vi "update GUI KF tuning.vi"(10 "Supervisor in":refnum<class "Supervisor.lvclass">, 11 "Vessel in":refnum<class "Vessel.lvclass">) -> (2 "Supervisor":refnum<class "Supervisor.lvclass">)   [LabVIEW 2014]
uses:
  ROV/Vessel.lvclass
  Supervisor/Supervisor.lvclass
  <vilib>/Analysis/Matrix/Datatypes/RealMatrix.ctl
  Observer/Kalman Filter/Kalman Filter.lvclass
  <vilib>/Analysis/Matrix/NI_Matrix.lvlib
panel:
  out "Real Matrix":T1
  in  "Name":string
  in  "Update Q":bool
  in  "Update R":bool
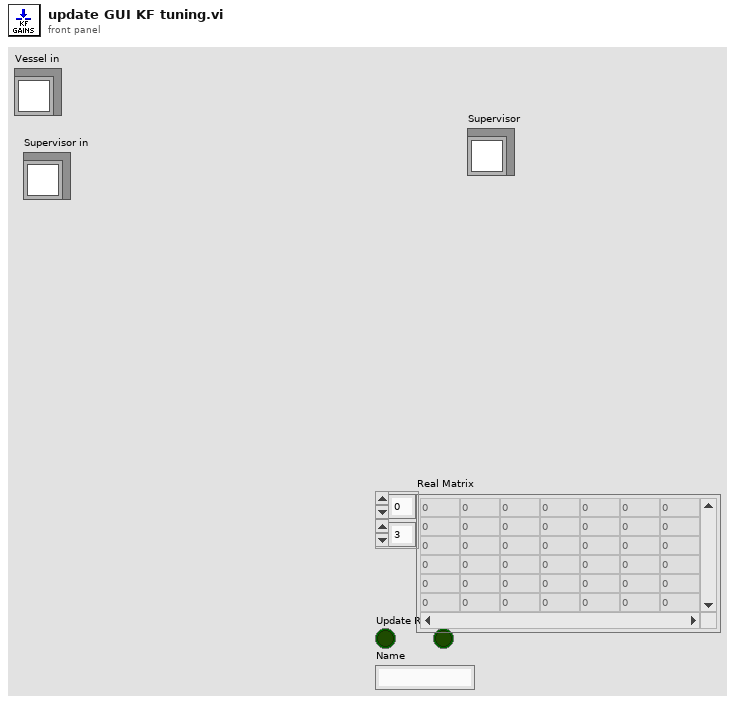
[diagram p1: front panel]
types:
  T1 = typedef "NI_Matrix.lvlib/RealMatrix.ctl" = dbl[][]
  T2 = cluster{"Real Matrix":T1, "Real Matrix":T1, "Update R":bool, "Update Q":bool, "Name":string}
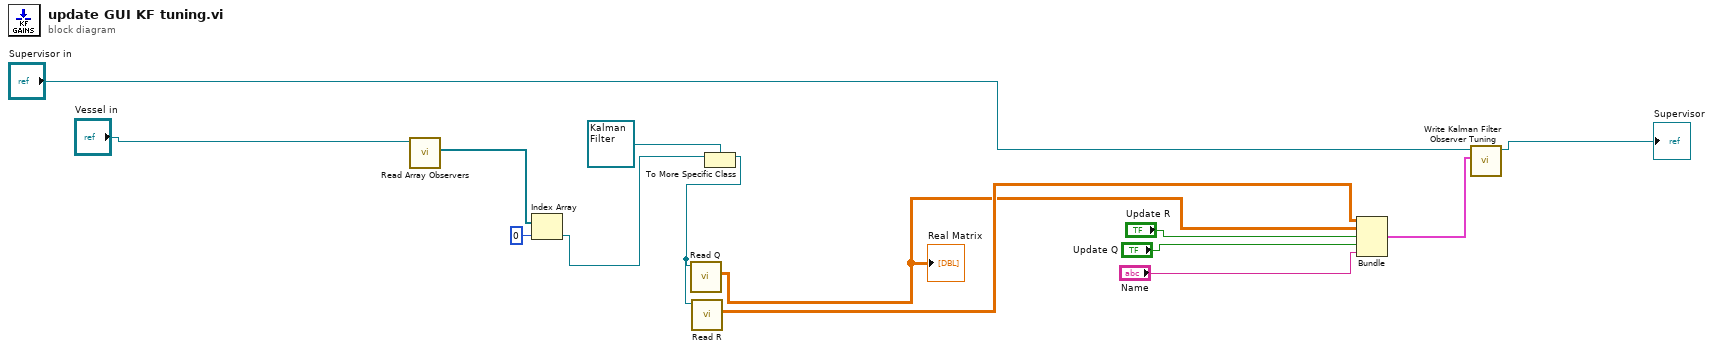
[diagram p0: block diagram]
diagram:
  n1 = call-dynamic "Read Array Observers.vi"("Vessel in"="Vessel in") -> ("Array Observers"=w13:refnum<class "Observer.lvclass">[])  [unwired: 8 in, 2 out]
  n2 = Index Array(array=w13, index=0) -> (element=w10:refnum<class "Observer.lvclass">)
  n3 = To More Specific Class(target class=refnum<class "Kalman Filter.lvclass"> refnum ("Observer Library.lvlib:Kalman Filter.lvclass"), reference=w10) -> (specific class reference=w9:refnum<class "Kalman Filter.lvclass">)  [unwired: 1 in, 1 out]
  n4 = call-dynamic "Read Q.vi"("Kalman Filter in"=w9) -> ("Real Matrix"=w3:T1)  [unwired: 8 in, 2 out]
  "Real Matrix" <- w3
  n5 = call-dynamic "Read R.vi"("Kalman Filter in"=w9) -> ("Real Matrix"=w4:T1)  [unwired: 8 in, 2 out]
  n6 = Bundle("Real Matrix"=w4, "Real Matrix"=w3, "Update R"="Update R", "Update Q"="Update Q", "Name"="Name") -> (w2:T2)  [unwired: 1 in]
  n7 = call-dynamic "Write Kalman Filter Observer Tuning.vi"("Kalman Filter Observer Tuning"=w2, "Supervisor in"="Supervisor in") -> ("Supervisor out"=→"Supervisor":refnum<class "Supervisor.lvclass">)  [unwired: 8 in, 1 out]
